vi "air flow.vi"(4 "State":i16, 5 "Time":dbl format="%.2f", 6 "Sensor Values":dbl[](array[numeric])=[120000.0, 10000.0], 7 "Set Points":dbl[](array[numeric])=[1.0, 22.0, 5e-05]) -> (0 "required data":T1={"Set Point names"=["accumulator volume (L)", "air temperature (C)", "air flow (M/s)"], "required number of setpoints"=3, "required number of sensors"=2, "Sensor names"=["Source pressure (Pa)", "Accumulator pressure (Pa)"]}, 3 "fraction on":dbl)   [LabVIEW 2010]
uses:
  <vilib>/Analysis/NI_AALPro.lvlib
panel:
  # "Enter the correct information for this control code in the required data structure below. Then make the current value default by right clicking on the border of the data structure."
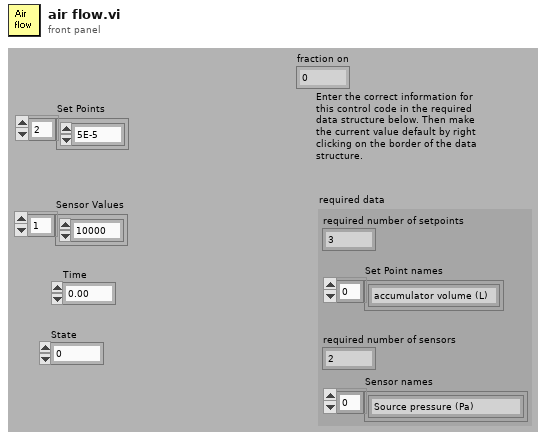
[diagram p1: front panel]
types:
  T1 = cluster{"Set Point names":string[], "required number of setpoints":u8, "required number of sensors":u8, "Sensor names":string[]}
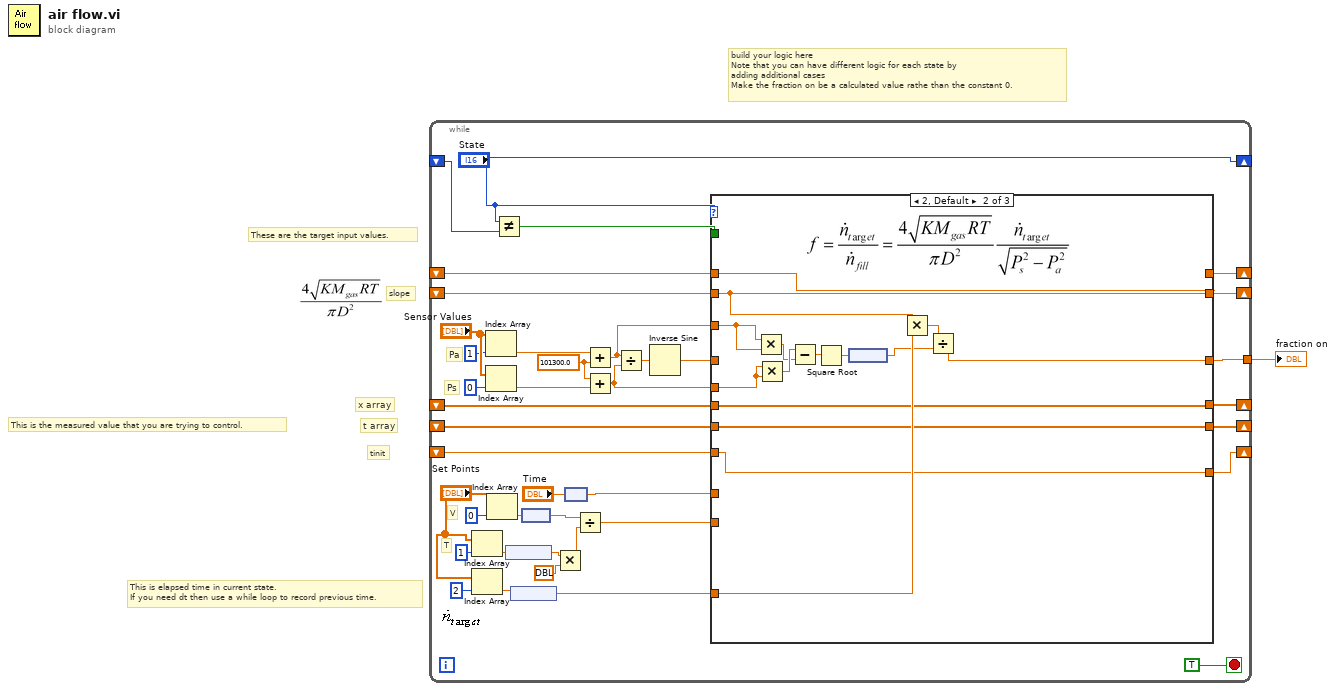
[diagram p0: block diagram]
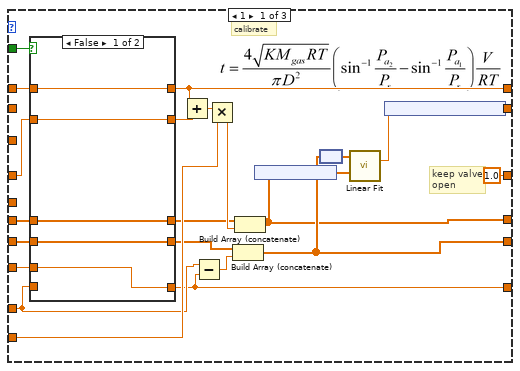
[diagram p2: hidden frame]
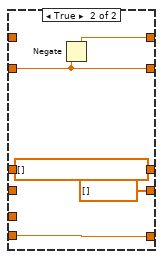
[diagram p3: hidden frame]
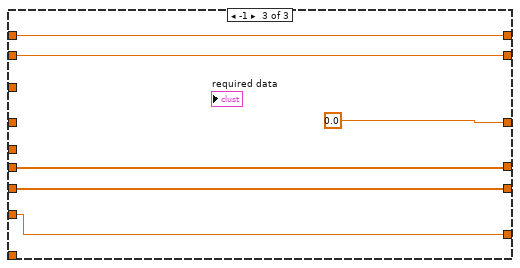
[diagram p4: hidden frame]
diagram:
  # "slope"
  # "tinit"
  # "t array"
  # "x array"
  # "build your logic here\nNote that you can have different logic for each state by\nadding additional cases\nMake the fraction on be a calculated value rathe than the constant 0."
  # "These are the target input values."
  # "This is the measured value that you are trying to control."
  # "This is elapsed time in current state.\nIf you need dt then use a while loop to record previous time."
  n1 = while {
    tunnel: [w41] -> w1
    shift-right: ["State"] -> _
    shift-left: _ -> [w37]
    shift-right: [w34] -> _
    shift-left: _ -> [w33]
    shift-right: [w20] -> _
    shift-left: _ -> [w21]
    shift-right: [w18] -> _
    shift-left: _ -> [w19]
    shift-right: [w16] -> _
    shift-left: _ -> [w15]
    shift-right: [w14] -> _
    shift-left: _ -> [w13]
    stop <- TRUE stop-if-true
    w2 = 101300.0 ("y")
    # "T"
    # "V"
    # "Ps"
    # "Pa"
    n2 = Index Array(array="Set Points", index=1) -> (element=w28:dbl)
    n3 = Index Array(array="Set Points", index=2) -> (element=w9:dbl)
    n4 = Index Array(array="Sensor Values", index=1) -> (element=w6:dbl)
    n5 = Index Array(array="Sensor Values", index=0) -> (element=w5:dbl)
    n6 = Index Array(array="Set Points", index=0) -> (element=w29:dbl)
    n7 = Not Equal?(x="State", y=w37) -> (x != y?=w35:bool)
    n8 = node(w28) -> (w26:dbl[unit])
    n9 = node(w9) -> (w8:dbl[unit])
    n10 = node(w29) -> (w27:dbl[unit])
    n11 = Multiply(x=w26, y=ext[unit] 8.314472) -> (x*y=w24:ext[unit])
    n12 = node("Time") -> (w17:dbl[unit])
    n13 = Divide(x=w27, y=w24) -> (x/y=w23:ext[unit])
    n14 = Add(x=w6, y=w2) -> (x+y=w3:dbl)
    n15 = Add(x=w2, y=w5) -> (x+y=w4:dbl)
    n16 = Divide(x=w3, y=w4) -> (x/y=w32:dbl)
    n17 = Inverse Sine(1:w32) -> (0:w31:dbl)
    n18 = case shown="2, Default" "State" {
      tunnel: [1.0 ("fraction on") w75 0.0 ("fraction on")] -> w41
      tunnel: w35 -> [w63 _ _]
      tunnel: w31 -> [w62 _ _]
      tunnel: [w60 w79 w93] -> w34
      tunnel: w33 -> [w61 w79 w93]
      tunnel: w23 -> [w58 _ _]
      tunnel: w17 -> [w48 _ _]
      tunnel: w21 -> [w54 w78 w92]
      tunnel: [w50 w78 w92] -> w20
      tunnel: w19 -> [w52 w77 w91]
      tunnel: [w51 w77 w91] -> w18
      tunnel: [w47 w76 w90] -> w16
      tunnel: w15 -> [w49 w76 w90]
      tunnel: [w45 w80 w94] -> w14
      tunnel: w13 -> [_ w80 w94]
      tunnel: w8 -> [_ w89 _]
      tunnel: w3 -> [_ w88 _]
      tunnel: w4 -> [_ w87 _]
      frame 1 {
        # "keep valve\nopen"
        # "calibrate"
        n19 = case shown="False" w63 {
          tunnel: w62 -> [w68 w73]
          tunnel: [w69 w74] -> w60
          tunnel: w61 -> [w69 _]
          tunnel: [w68 w73] -> w57
          tunnel: [w67 ext[unit][] []] -> w55
          tunnel: w54 -> [w67 _]
          tunnel: [w66 dbl[unit][] []] -> w53
          tunnel: w52 -> [w66 _]
          tunnel: [w65 w70] -> w47
          tunnel: w48 -> [_ w70]
          tunnel: w49 -> [w65 _]
          frame False {
          }
          frame True {
            n20 = Negate(x=w73) -> (-x=w74:dbl)
          }
        }
        n21 = Add(x=w60, y=w57) -> (x+y=w59:dbl)
        n22 = Subtract(x=w48, y=w47) -> (x-y=w46:dbl[unit])
        n23 = Multiply(x=w59, y=w58) -> (x*y=w56:ext[unit])
        n24 = Build Array (concatenate)(w53, w46) -> (w51:dbl[unit][])
        n25 = Build Array (concatenate)(w55, w56) -> (w50:ext[unit][])
        n26 = node(w50) -> (w43:ext[])
        n27 = node(w51) -> (w44:dbl[])
        n28 = call <vilib>:"Linear Fit.vi"("Y"=w44, "X"=w43) -> ("slope"=w42:dbl)  [unwired: 9 in, 4 out]
        n29 = node(w42) -> (w45:dbl[unit])
      }
      frame 2, Default {
        n30 = Multiply(x=w88, y=w88) -> (x*y=w85:dbl)
        n31 = Multiply(x=w87, y=w87) -> (x*y=w86:dbl)
        n32 = Subtract(x=w86, y=w85) -> (x-y=w84:dbl)
        n33 = Square Root(x=w84) -> (sqrt(x)=w83:dbl)
        n34 = node(w83) -> (w81:dbl[unit])
        n35 = Multiply(x=w80, y=w89) -> (x*y=w82:dbl[unit])
        n36 = Divide(x=w82, y=w81) -> (x/y=w75:dbl)
      }
      frame -1 {
      }
    }
  }
  "fraction on" <- w1
